vi "Main - Json Status.vi"(11 "json":string="{\"status\":\"error\",\"message\":\"No records found for fileid: 6\"}") -> (3 "Success?":bool, 5 "message":string)   [LabVIEW 2019]
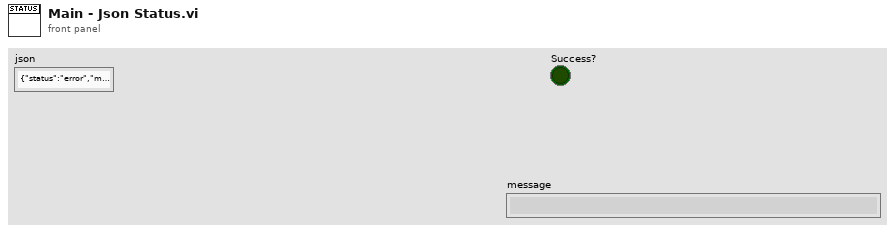
[diagram p1: front panel]
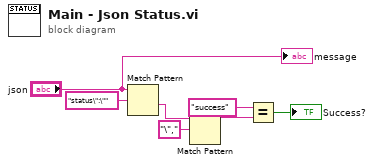
[diagram p0: block diagram]
diagram:
  n1 = Match Pattern(string="json", regular expression="status\":\"") -> (after substring=w6:string)  [unwired: 1 in, 3 out]
  n2 = Match Pattern(string=w6, regular expression="\",") -> (before substring=w4:string)  [unwired: 1 in, 3 out]
  n3 = Equal?(x="success", y=w4) -> (x = y?=→"Success?":bool)
  "message" <- "json"
